vi "Eval_SglRes.vi"(8 "error in (no error)":errorcluster, 11 "muExpr in":refnum<class "mupExpr.lvclass">) -> (0 "error out":errorcluster, 2 "Result":dbl format="%#_13g", 3 "muExpr out":refnum<class "mupExpr.lvclass">)   [LabVIEW 2015, in "mupExpr.lvclass"]
doc: "Evaluate the expression and return a single result.\n\nIf multiple expressions have been input, the result of the last one in the list is returned.\n\nIf the variables are defined for bulk mode evaluation, only the first set (index 0) will be evaluated."
uses:
  mupExpr.lvclass
  mupExpr.lvclass/mupExpr.ctl
  mupLib/mupCheckError.vi
  <vilib>/Utility/error.llb/Error Cluster From Error Code.vi
  mupLib/mupLib.lvlib
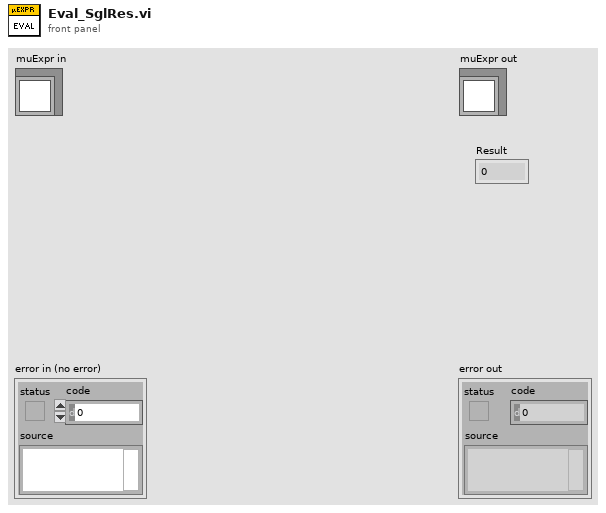
[diagram p1: front panel]
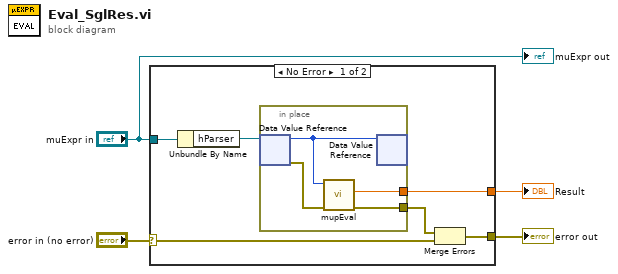
[diagram p0: block diagram]
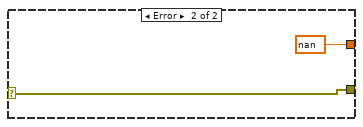
[diagram p2: hidden frame]
diagram:
  n1 = case shown="No Error" "error in (no error)" {
    selector: "error in (no error)" -> [w6 w16]
    tunnel: [w7 w16] -> w4
    tunnel: "muExpr in" -> [w5 _]
    tunnel: [w10 nan ("result")] -> w3
    frame No Error {
      n2 = Unbundle By Name(w5) -> ("hParser"=w9:refnum<data-value>)
      n3 = in-place {
        in-place-border: [w14] -> w8
        in-place-border: [w13] -> w10
        n4 = in-place-dvr #1(w9) -> (w12:u64, w11:errorcluster)
        n5 = call "mupEval.vi"("error in (no error)"=w11, "hParser in"=w12) -> ("error out"=w14:errorcluster, "result"=w13:dbl)  [unwired: 7 in, 1 out]
        n6 = in-place-dvr #1(w12) -> ()  [unwired: 2 out]
      }
      n7 = Merge Errors(w8, w6) -> (w7:errorcluster)
    }
    frame Error {
    }
  }
  "error out" <- w4
  "Result" <- w3
  "muExpr out" <- "muExpr in"
